vi "Set Default.vi"(1 "VI引用":refnum<vi>) -> (0 "引用输出":refnum<vi>)   [LabVIEW 2018]
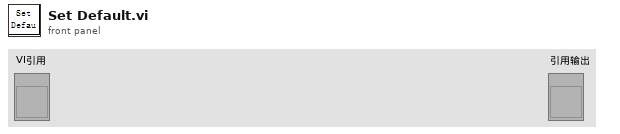
[diagram p1: front panel]
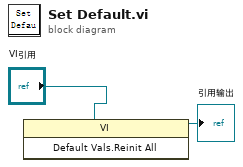
[diagram p0: block diagram]
diagram:
  n1 = invoke class="VI" method="Default Vals.Reinit All"(reference="VI引用") -> (reference out=→"引用输出":refnum<vi>)  [unwired: 2 in, 2 out]
